vi "Search_for_MDrive.vi"(1 "Port Name":string) -> ()   [LabVIEW 2010]
panel:
  out "FoundDrives":cluster{i32, "String Reply":string}[](array[cluster])
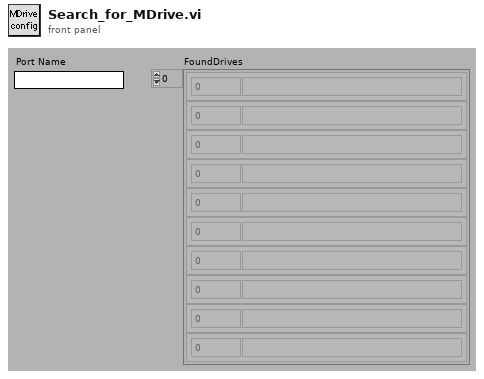
[diagram p1: front panel]
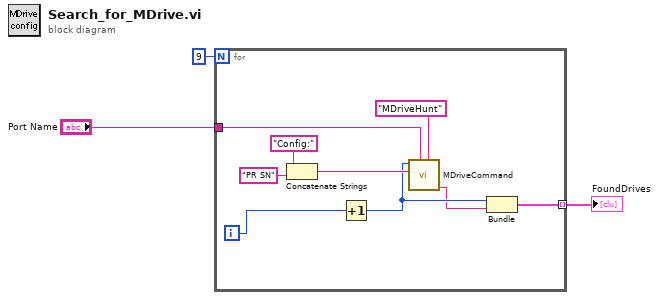
[diagram p0: block diagram]
diagram:
  n1 = for {
    N: 9 -> [_]
    tunnel: [w5] -> w1 mode=indexing
    tunnel: "Port Name" -> [w4]
    i -> [w9]
    n2 = Concatenate Strings("Config:" ("string"), "PR SN" ("string")) -> (w11:string)
    n3 = Increment(x=w9) -> (x+1=w7:i32)
    n4 = call "MDriveCommand.vi"("Channel Name"="MDriveHunt", "Port Name"=w4, "MDriveCommand"=w11, "Address"=w7) -> ("String Reply"=w6:string)  [unwired: 1 in, 5 out]
    n5 = Bundle(w7, "String Reply"=w6) -> (w5:cluster{i32, "String Reply":string})  [unwired: 1 out]
  }
  "FoundDrives" <- w1
